vi "build tree table in CSM-VI mode.vi"(6 "Config Path":path, 8 "Error In":errorcluster caption="Error in (no error)", 9 "Option":T1) -> (0 "Error Out":errorcluster, 2 "Type":string[](array[string]), 3 "Tree Table":string[][](array[string]))   [LabVIEW 2017, in "interfacebrowser.lvlib"]
uses:
  interfacebrowser.lvlib
  _csmHelper/API with lvcsm Support/CSM-Helper API with lvcsm Support.lvlib
  Communicable State Machine.lvlib
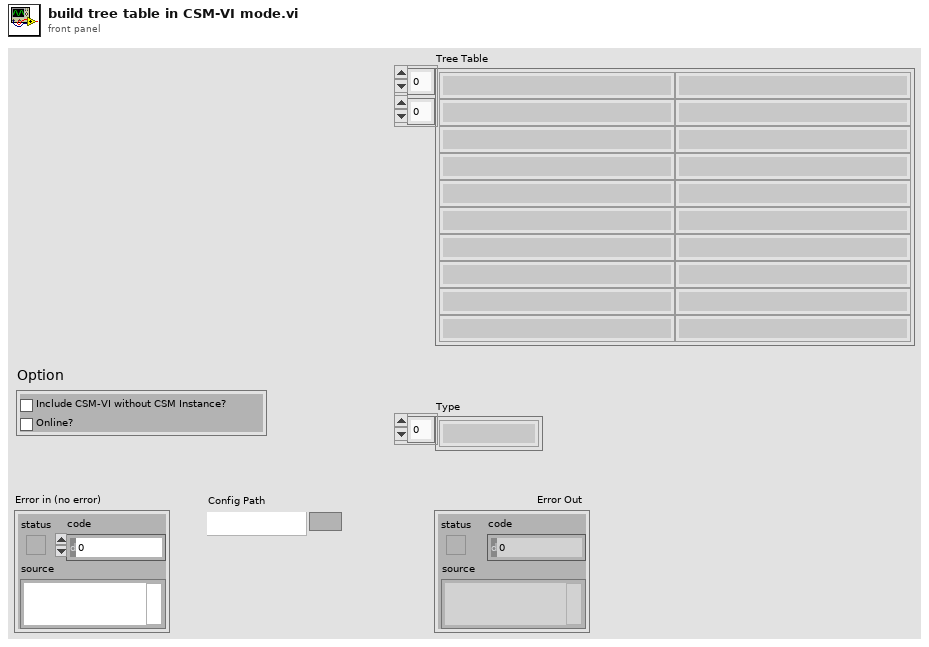
[diagram p1: front panel]
types:
  T1 = cluster{"Opton:All-CSM-VIs":bool, "Option:Online Only":bool}
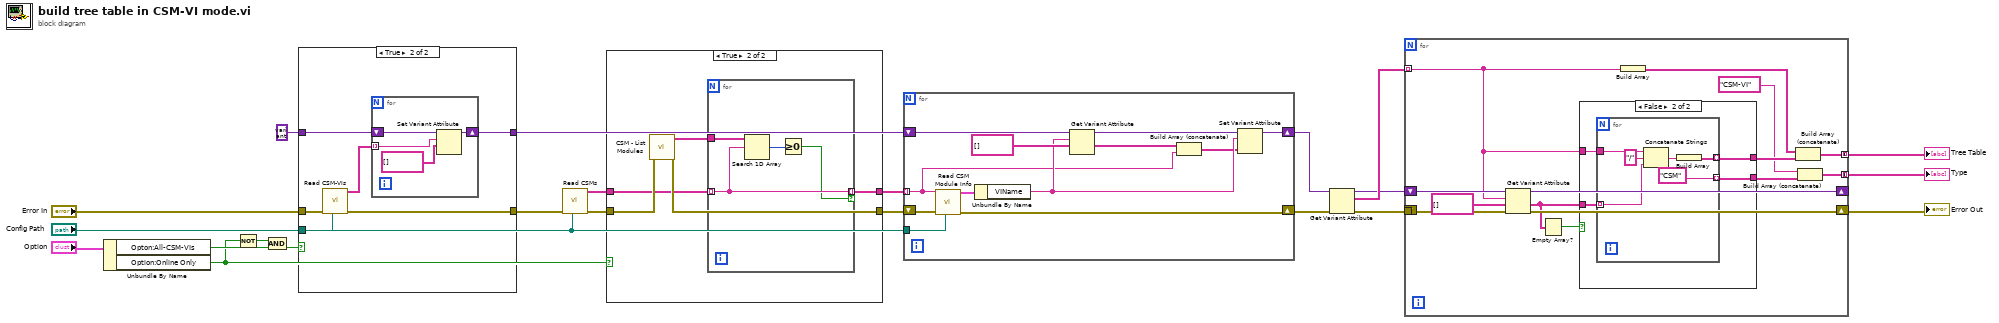
[diagram p0: block diagram]
diagram:
  n1 = Unbundle By Name("Option") -> ("Opton:All-CSM-VIs"=w7:bool, "Option:Online Only"=w2:bool)
  n2 = Not(x=w2) -> (.not. x?=w1:bool)
  n3 = And(x=w1, y=w7) -> (x .and. y?=w3:bool)
  n4 = case shown="True" w3 {
    tunnel: "Error In" -> [w24 w30]
    tunnel: [w24 w29] -> w12
    tunnel: variant -> [w23 w28]
    tunnel: [w23 w27] -> w10
    tunnel: "Config Path" -> [_ w25]
    frame False {
    }
    frame True {
      n5 = call "Read CSM-VIs.vi"("Config Path"=w25, "Error In"=w30) -> ("Error Out"=w29:errorcluster, "Array"=w26:string[])  [unwired: 8 in]
      n6 = for {
        shift-right: [w33] -> w27
        shift-left: w28 -> [w34]
        tunnel: w26 -> [w31] mode=indexing
        n7 = Set Variant Attribute(Variant=w34, name=w31, value=string[] [] ("Delimiter")) -> (Variant out=w33:variant)  [unwired: 1 in, 2 out]
      }
    }
  }
  n8 = call "Read CSMs.vi"("Config Path"="Config Path", "Error In"=w12) -> ("Error Out"=w21:errorcluster, "Array"=w4:string[])  [unwired: 8 in]
  n9 = case shown="True" w2 {
    tunnel: w21 -> [w35 w41]
    tunnel: [w35 w40] -> w6
    tunnel: [w36 w37] -> w5
    tunnel: w4 -> [w36 w38]
    frame False {
    }
    frame True {
      n10 = call "CSM - List Modules.vi"("Error In"=w41) -> ("error out"=w40:errorcluster, "Module Names"=w39:string[])  [unwired: 9 in]
      n11 = for {
        tunnel: w39 -> [w45]
        tunnel: w38 -> [w44] mode=indexing
        tunnel: [w44] -> w37 mode=indexing if=w42
        n12 = Search 1D Array(1D array=w45, element=w44) -> (index of element=w43:i32)  [unwired: 1 in]
        n13 = Greater Or Equal To 0?(x=w43) -> (x >= 0?=w42:bool)
      }
    }
  }
  n14 = for {
    tunnel: w5 -> [w46] mode=indexing
    tunnel: "Config Path" -> [w55]
    shift-right: [w54] -> w20
    shift-left: w6 -> [w56]
    shift-right: [w50] -> w19
    shift-left: w10 -> [w53]
    n15 = call "Read CSM Module Info.vi"("Config Path"=w55, "error in (no error)"=w56, "CSM Name"=w46) -> ("error out"=w54:errorcluster, "Cluster"=w57:cluster{"VIName":string})  [unwired: 7 in]
    n16 = Unbundle By Name(w57) -> ("VIName"=w49:string)
    n17 = Get Variant Attribute(Variant=w53, name=w49, default value (empty Variant)=string[] [] ("Delimiter")) -> (duplicate Variant=w51:variant, value=w48:string[])  [unwired: 1 in, 2 out]
    n18 = Build Array (concatenate)(w48, w46) -> (w47:string[])
    n19 = Set Variant Attribute(Variant=w51, name=w49, value=w47) -> (Variant out=w50:variant)  [unwired: 1 in, 2 out]
  }
  n20 = Get Variant Attribute(Variant=w19, error in=w20) -> (duplicate Variant=w17:variant, names=w18:string[], error out=w16:errorcluster)  [unwired: 2 in, 1 out]
  n21 = for {
    tunnel: w18 -> [w65] mode=indexing
    shift-right: [w69] -> _
    shift-left: w17 -> [w70]
    tunnel: w16 -> [w68]
    shift-right: [w67] -> w15
    shift-left: _ -> [_]
    tunnel: [w64] -> w14 mode=concatenating
    tunnel: [w62] -> w13 mode=concatenating
    n22 = Get Variant Attribute(Variant=w70, name=w65, default value (empty Variant)=string[] [] ("Delimiter"), error in=w68) -> (duplicate Variant=w69:variant, value=w59:string[], error out=w67:errorcluster)  [unwired: 1 out]
    n23 = Empty Array?(array=w59) -> (empty?=w58:bool)
    n24 = case shown="False" w58 {
      tunnel: [_ w75] -> w66
      tunnel: w65 -> [_ w74]
      tunnel: [_ w73] -> w61
      tunnel: w59 -> [_ w72]
      frame True {
      }
      frame False {
        n25 = for {
          tunnel: w74 -> [w81]
          tunnel: w72 -> [w80] mode=indexing
          tunnel: [w77] -> w75 mode=indexing
          tunnel: ["CSM" ("string")] -> w73 mode=indexing
          n26 = Concatenate Strings(w81, "/" ("string"), w80) -> (w78:string)
          n27 = Build Array(w78) -> (w77:string[])
        }
      }
    }
    n28 = Build Array(w65) -> (w63:string[])
    n29 = Build Array (concatenate)(w63, w66) -> (w64:string[][])
    n30 = Build Array (concatenate)("CSM-VI" ("string"), w61) -> (w62:string[])
  }
  "Type" <- w13
  "Tree Table" <- w14
  "Error Out" <- w15
